vi "Get VI Advanced Metrics(冲突时的文件备份2013-05-03 10-48-04).vi"() -> ()   [LabVIEW 2012]
panel:
  out "Metrics:Advanced":T1
  in  "停止按钮":bool
  out "VI Metrics":T2
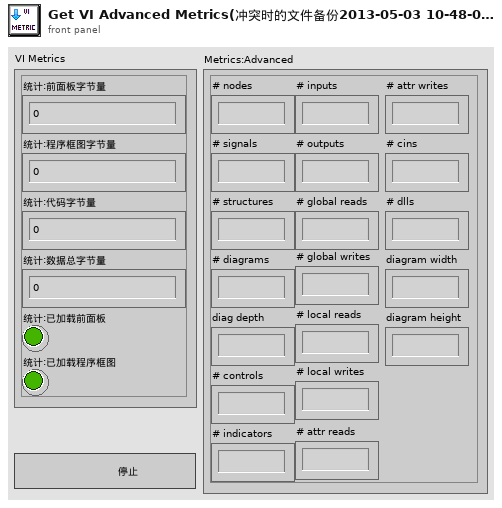
[diagram p1: front panel]
types:
  T1 = cluster{"# nodes":u32, "# signals":u32, "# structures":u32, "# diagrams":u32, "diag depth":u32, "# controls":u32, "# indicators":u32, "# inputs":u32, "# outputs":u32, "# global reads":u32, "# global writes":u32, "# local reads":u32, "# local writes":u32, "# attr reads":u32, "# attr writes":u32, "# cins":u32, "# dlls":u32, "diagram width":u32, "diagram height":u32}
  T2 = cluster{"统计:前面板字节量":u32, "统计:程序框图字节量":u32, "统计:代码字节量":u32, "统计:数据总字节量":u32, "统计:已加载前面板":bool, "统计:已加载程序框图":bool}
  T3 = cluster{"Metric.FPSize":u32, "Metric.BDSize":u32, "Metric.CodeSize":u32, "Metric.DataSize":u32, "PanelLoaded":bool, "DiagramLoaded":bool}
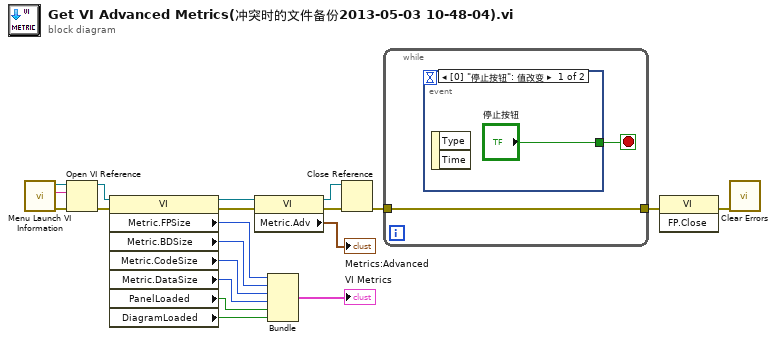
[diagram p0: block diagram]
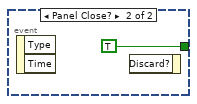
[diagram p2: hidden frame]
diagram:
  n1 = call <vilib>:"Menu Launch VI Information.vi"() -> ("error out"=w18:errorcluster, "Menu Launch:VI"=w20:string, "Menu Launch:App"=w19:refnum<vi>)  [unwired: 9 in]
  n2 = Open VI Reference(application reference (local)=w19, vi path=w20, error in (no error)=w18) -> (vi reference=w17:refnum<vi>, error out=w16:errorcluster)  [unwired: 3 in]
  n3 = property class="VI"(reference=w17, error in=w16) -> (reference out=w4:refnum<vi>, error out=w5:errorcluster, "Metric.FPSize"=w14:u32, "Metric.BDSize"=w13:u32, "Metric.CodeSize"=w12:u32, "Metric.DataSize"=w11:u32, "PanelLoaded"=w10:bool, "DiagramLoaded"=w9:bool)
  n4 = property class="VI"(reference=w4, error in=w5) -> (reference out=w2:refnum<vi>, error out=w3:errorcluster, "Metric.Adv"=→"Metrics:Advanced":T1)
  n5 = Bundle("Metric.FPSize"=w14, "Metric.BDSize"=w13, "Metric.CodeSize"=w12, "Metric.DataSize"=w11, "PanelLoaded"=w10, "DiagramLoaded"=w9) -> (→"VI Metrics":T3)  [unwired: 1 in]
  n6 = Close Reference(reference=w2, error in (no error)=w3) -> (error out=w8:errorcluster)
  n7 = while {
    tunnel: w8 -> [w21]
    tunnel: [w21] -> w7
    stop <- w22 stop-if-true
    n8 = event shown="[0] \"停止按钮\": 值改变" {
      selector: _ -> [_ _]
      dyn-events: _ -> [_ _]
      timeout: _ -> [_ _]
      tunnel: ["停止按钮" TRUE ("停止按钮")] -> w22
      event "停止按钮": Value Change {
        n9 = event-data() -> ()  [unwired: 1 in, 2 out]
      }
      event Panel Close? {
        n10 = event-data() -> ()  [unwired: 1 in, 2 out]
        n11 = event-data() -> ()  [unwired: 2 in, 1 out]
      }
    }
  }
  n12 = invoke class="VI" method="FP.Close"(error in=w7) -> (error out=w6:errorcluster)  [unwired: 2 in, 2 out]
  n13 = call <vilib>:"Clear Errors.vi"("error in (no error)"=w6) -> ()  [unwired: 6 in, 1 out]
